vi "test_scope_read.vi"() -> ()   [LabVIEW 2011]
uses:
  scope/Agilent_546XX_Series/Agilent 546XX Series.lvlib
panel:
  in  "Time Delay":dbl=1.5
  in  "Holdoff Time":dbl=0.001
  in  "Voltage Range":dbl
  in  "Time Range":dbl
  in  "Trigger Coupling":u32(slide) scale=0.0..1.0
  in  "Channel Select":u32(slide) scale=1.0..2.0
  in  "Trigger Level":dbl
  in  "Capture Mode":string(combo)="Run"
  out "'Scope Data":cluster{"Y":dbl[], "Y":dbl[]}[](graph)
  in  "VISA Boonton In":refnum<visa-resource-name>
  in  "Boonton Data":path
  in  "Boonton Commands":path
  in  "Scope Data":path
  out "error out":errorcluster {"code" format="%.0x"}
  in  "error in (no error)":errorcluster {"code" format="%.0x"}
  in  "VISA Scope In":refnum<visa-resource-name>
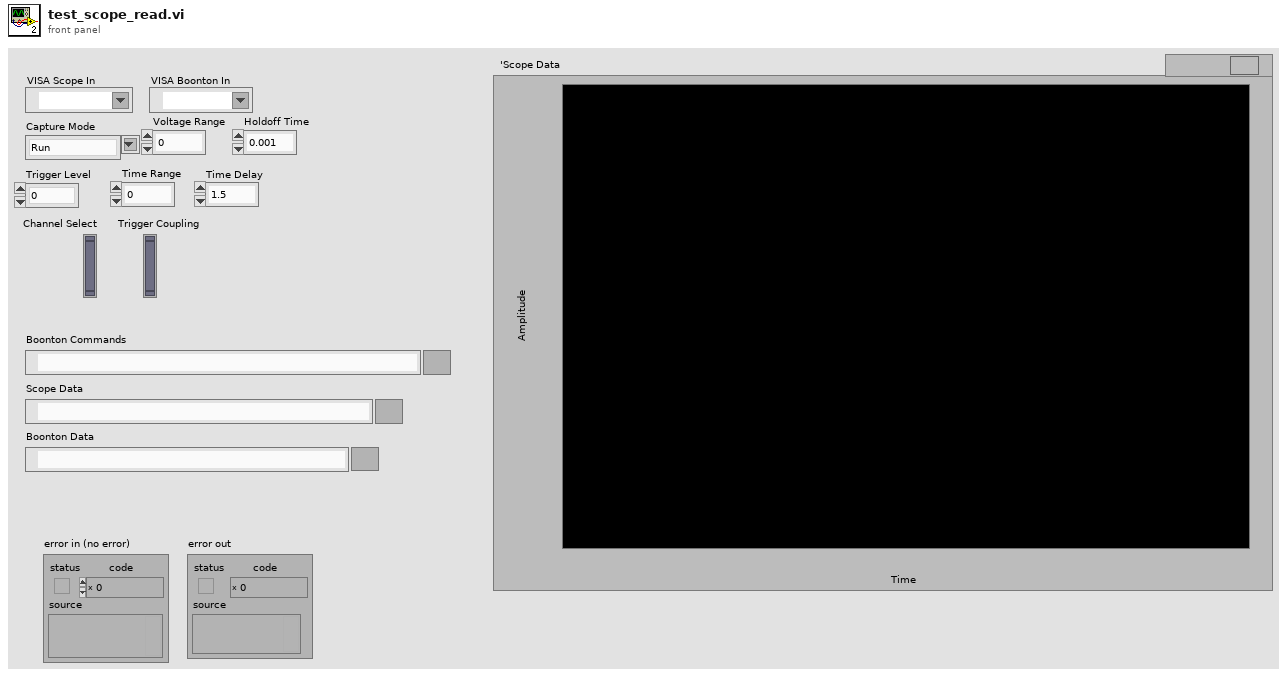
[diagram p1: front panel]
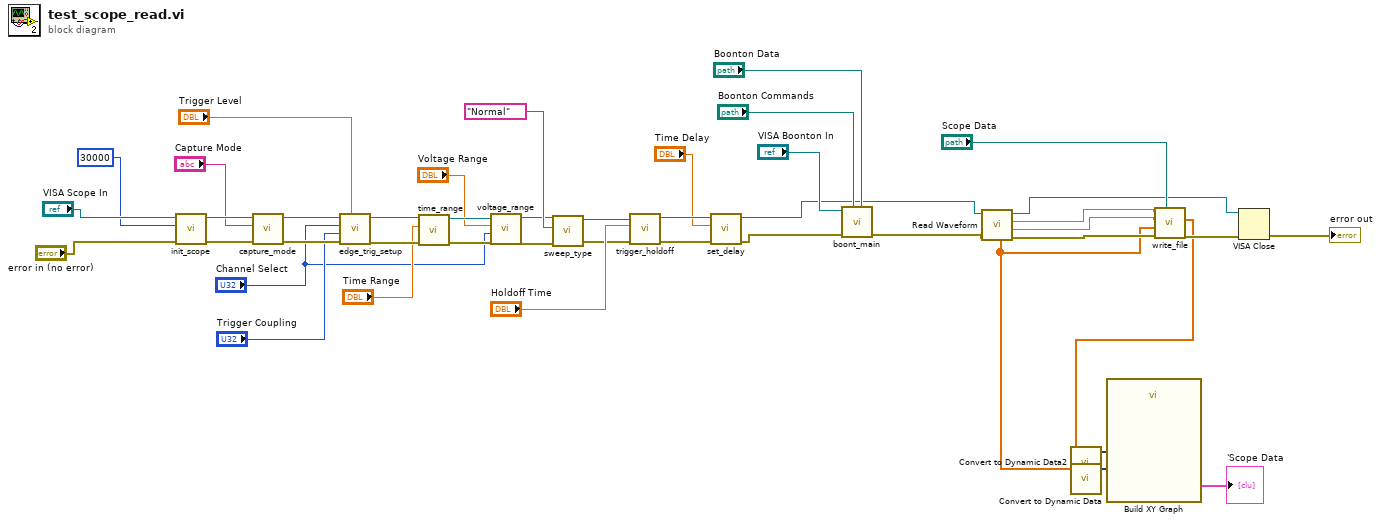
[diagram p0: block diagram]
diagram:
  n1 = call "init_scope.vi"("error in (no error)"="error in (no error)", "VISA Timeout (millis)"=30000, "VISA Scope"="VISA Scope In") -> ("error out"=w30:errorcluster, "VISA Scope Out"=w31:refnum<visa-resource-name>)  [unwired: 7 in]
  n2 = call "capture_mode.vi"("error in (no error)"=w30, "Capture Mode"="Capture Mode", "VISA In"=w31) -> ("error out"=w27:errorcluster, "VISA Out"=w28:refnum<visa-resource-name>)  [unwired: 7 in]
  n3 = call "edge_trig_setup.vi"("Tigger Level"="Trigger Level", "error in (no error)"=w27, "Coupling"="Trigger Coupling", "Channel"="Channel Select", "VISA In"=w28) -> ("error out"=w23:errorcluster, "VISA Out"=w24:refnum<visa-resource-name>)  [unwired: 5 in]
  n4 = call "time_range.vi"("error in (no error)"=w23, "Time Range"="Time Range", "VISA In"=w24) -> ("error out"=w14:errorcluster, "VISA Out"=w15:refnum<visa-resource-name>)  [unwired: 7 in]
  n5 = call "voltage_range.vi"("error in (no error)"=w14, "Channel Select"="Channel Select", "Voltage"="Voltage Range", "VISA In"=w15) -> ("error out"=w2:errorcluster, "VISA Out"=w5:refnum<visa-resource-name>)  [unwired: 6 in]
  n6 = call "sweep_type.vi"("error in (no error)"=w2, "Sweep Type"="Normal", "VISA In"=w5) -> ("error out"=w3:errorcluster, "VISA Out"=w4:refnum<visa-resource-name>)  [unwired: 7 in]
  n7 = call "trigger_holdoff.vi"("error in (no error)"=w3, "Holdoff Time"="Holdoff Time", "VISA Scope In"=w4) -> ("error out"=w10:errorcluster, "VISA Out"=w9:refnum<visa-resource-name>)  [unwired: 6 in]
  n8 = call "set_delay.vi"("error in (no error)"=w10, "Delay"="Time Delay", "VISA Scope In"=w9) -> ("error out"=w1:errorcluster, "VISA Out"=w7:refnum<visa-resource-name>)  [unwired: 7 in]
  n9 = call "boont_main.vi"("Data File"="Boonton Data", "Command File"="Boonton Commands", "error in (no error)"=w1, "VISA In"="VISA Boonton In") -> ("error out"=w20:errorcluster)  [unwired: 6 in, 1 out]
  n10 = call "Read Waveform.vi"("error in (no error)"=w20, "VISA Resource Name"=w7) -> ("error out"=w21:errorcluster, "x increment"=w16:dbl, "initial x"=w17:dbl, "VISA Resource Name Out"=w18:refnum<visa-resource-name>, "waveform array"=w19:dbl[])  [unwired: 4 in, 1 out]
  n11 = call "Convert to Dynamic Data"("Array"=w19) -> ("Dynamic Data Type"=w37:dynamicdata)  [unwired: 3 in]
  n12 = call "write_file.vi"("Data File"="Scope Data", "error in (no error)"=w21, "Y Axis Data"=w19, "Step Size"=w16, "Initial Value"=w17) -> ("error out"=w43:errorcluster, "xArray"=w36:dbl[])  [unwired: 4 in]
  n13 = call "Convert to Dynamic Data2"("Array"=w36) -> ("Dynamic Data Type"=w35:dynamicdata)  [unwired: 3 in]
  n14 = call "Build XY Graph"("Y Input"=w37, "X Input"=w35) -> ("XY Graph"=→"'Scope Data":cluster{"Y":dbl[], "Y":dbl[]}[])  [unwired: 3 in, 6 out]
  n15 = VISA Close(VISA resource name=w18, error in (no error)=w43) -> (error out=→"error out":errorcluster)
